vi "Write Start hidden.vi"(8 "error in (no error)":errorcluster, 10 "Start hidden":bool, 11 "Fiber Auto Collimation panel in":refnum<class "Fiber Auto Collimation panel.lvclass">) -> (0 "error out":errorcluster, 3 "Fiber Auto Collimation panel out":refnum<class "Fiber Auto Collimation panel.lvclass">)   [LabVIEW 2018, in "Fiber Auto Collimation panel.lvclass"]
doc: "Tells the VI to start hidden or not. Usually this is False, as it's a panel and should be a \"pop-up\", but if this panel is going to be put inside a sub-panel then this should be True."
uses:
  Fiber Auto Collimation panel.lvclass
  Fiber Auto Collimation panel.lvclass/Fiber Auto Collimation panel.ctl
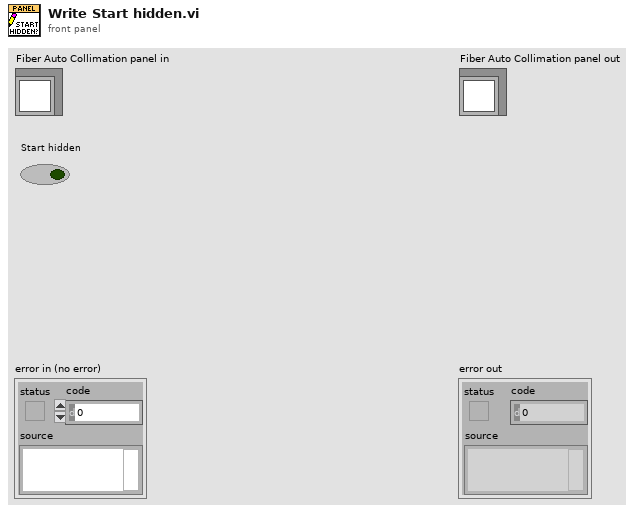
[diagram p1: front panel]
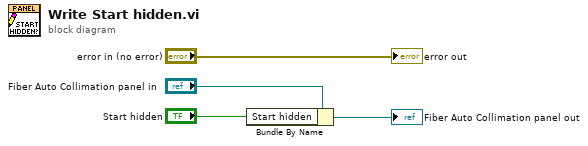
[diagram p0: block diagram]
diagram:
  n1 = Bundle By Name(cluster="Fiber Auto Collimation panel in", "Start hidden"="Start hidden") -> (→"Fiber Auto Collimation panel out":refnum<class "Fiber Auto Collimation panel.lvclass">)
  "error out" <- "error in (no error)"
